vi "DataManagementGetTrendPointsForDataEventResponse_Name.vi"() -> (1 "MessageName":string)   [LabVIEW 2017]
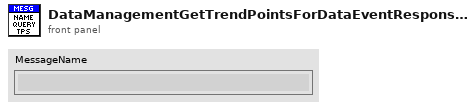
[diagram p1: front panel]
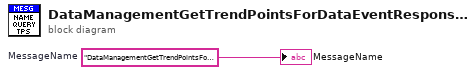
[diagram p0: block diagram]
diagram:
  w1 = "DataManagementGetTrendPointsForDataEventResponse"  # MessageName
  "MessageName" <- w1
